vi "Merge Results.vi"(4 "Result 2":T1={"Id"="", "Score"={"Status"=enum."Passed", "cpu_time"=-1, "max_memory"=-1, "style_score"=-1, "score0"="", "score1"="", "score2"="", "score3"="", "score4"="", "score5"=""}}, 5 "Results 1":T1={"Id"="", "Score"={"Status"=enum."Passed", "cpu_time"=-1, "max_memory"=-1, "style_score"=-1, "score0"="", "score1"="", "score2"="", "score3"="", "score4"="", "score5"=""}}) -> (1 "Results":T1={"Id"="", "Score"={"Status"=enum."Passed", "cpu_time"=-1, "max_memory"=-1, "style_score"=-1, "score0"="", "score1"="", "score2"="", "score3"="", "score4"="", "score5"=""}})   [LabVIEW 2013, in "VIChallenge.lvlib"]
doc: "This VI merges two results by selecting the worst case status, adding CPU times, selecting worst case memory usage, worst style score and concatenating custom score fields."
uses:
  <vilib>/LabVIEW Hacker/VIChallenge/VIChallenge.lvlib
  <vilib>/LabVIEW Hacker/VIChallenge/Private/Grader/Type Defs/Grader Result.ctl
  <vilib>/LabVIEW Hacker/VIChallenge/Private/Type Defs/Database/Score.ctl
  <vilib>/LabVIEW Hacker/VIChallenge/Private/Grader/Type Defs/UTF Status.ctl
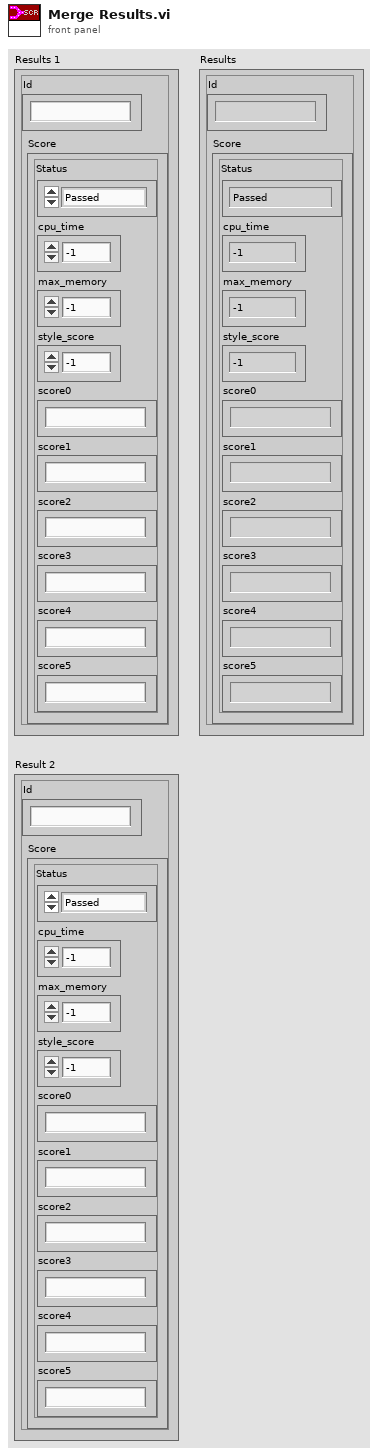
[diagram p1: front panel]
types:
  T1 = typedef "VIChallenge.lvlib/Grader Result.ctl" = cluster{"Id":string, "Score":T2}
  T2 = typedef "VIChallenge.lvlib/Score.ctl" = cluster{"Status":T3, "cpu_time":i32, "max_memory":i32, "style_score":i32, "score0":string, "score1":string, "score2":string, "score3":string, "score4":string, "score5":string}
  T3 = typedef "VIChallenge.lvlib/UTF Status.ctl" = enum16{"Null", "Passed", "Failed", "Error", "Skipped", "Not Processed"}
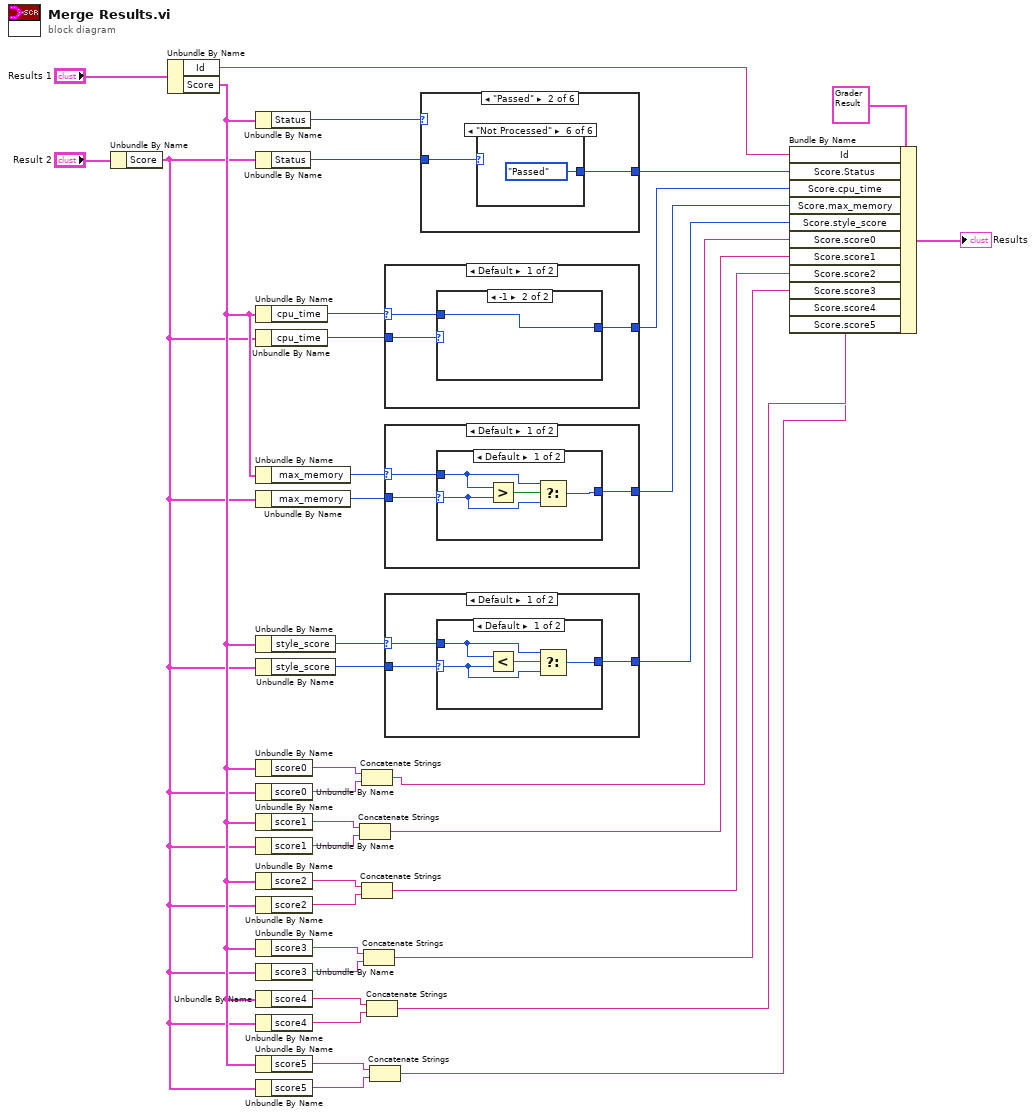
[diagram p0: block diagram]
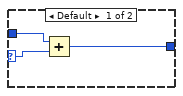
[diagram p6: hidden frame]
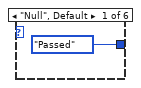
[diagram p9: hidden frame]
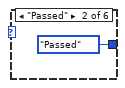
[diagram p10: hidden frame]
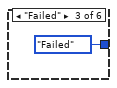
[diagram p11: hidden frame]
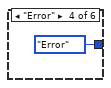
[diagram p12: hidden frame]
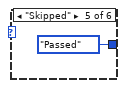
[diagram p13: hidden frame]
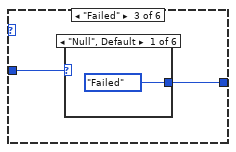
[diagram p14: hidden frame]
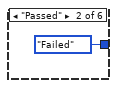
[diagram p15: hidden frame]
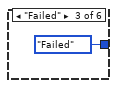
[diagram p16: hidden frame]
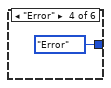
[diagram p17: hidden frame]
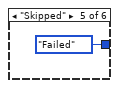
[diagram p18: hidden frame]
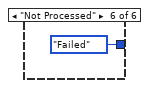
[diagram p19: hidden frame]
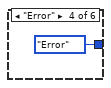
[diagram p20: hidden frame]
diagram:
  n1 = Unbundle By Name("Result 2") -> ("Score"=w14:T2)
  n2 = Unbundle By Name("Results 1") -> ("Id"=w35:string, "Score"=w15:T2)
  n3 = Unbundle By Name(w15) -> ("Status"=w34:T3)
  n4 = Unbundle By Name(w14) -> ("Status"=w32:T3)
  n5 = Unbundle By Name(w15) -> ("cpu_time"=w7:i32)
  n6 = Unbundle By Name(w14) -> ("cpu_time"=w29:i32)
  n7 = Unbundle By Name(w15) -> ("max_memory"=w5:i32)
  n8 = Unbundle By Name(w14) -> ("max_memory"=w4:i32)
  n9 = Unbundle By Name(w15) -> ("style_score"=w3:i32)
  n10 = Unbundle By Name(w14) -> ("style_score"=w2:i32)
  n11 = Unbundle By Name(w15) -> ("score0"=w28:string)
  n12 = Unbundle By Name(w14) -> ("score0"=w27:string)
  n13 = Unbundle By Name(w15) -> ("score1"=w24:string)
  n14 = Unbundle By Name(w14) -> ("score1"=w25:string)
  n15 = Unbundle By Name(w15) -> ("score2"=w23:string)
  n16 = Unbundle By Name(w14) -> ("score2"=w22:string)
  n17 = Unbundle By Name(w15) -> ("score3"=w20:string)
  n18 = Unbundle By Name(w14) -> ("score3"=w21:string)
  n19 = Unbundle By Name(w15) -> ("score4"=w19:string)
  n20 = Unbundle By Name(w14) -> ("score4"=w18:string)
  n21 = Unbundle By Name(w15) -> ("score5"=w16:string)
  n22 = Unbundle By Name(w14) -> ("score5"=w17:string)
  n23 = Concatenate Strings(w24, w25) -> (w13:string)
  n24 = Concatenate Strings(w28, w27) -> (w26:string)
  n25 = Concatenate Strings(w23, w22) -> (w12:string)
  n26 = Concatenate Strings(w20, w21) -> (w11:string)
  n27 = Concatenate Strings(w19, w18) -> (w10:string)
  n28 = Concatenate Strings(w16, w17) -> (w9:string)
  n29 = case shown="Default" w7 {
    selector: w7 -> [w38 _]
    tunnel: [w39 w45] -> w30
    tunnel: w29 -> [w40 w45]
    frame Default {
      n30 = case shown="-1" w40 {
        selector: w40 -> [w42 _]
        tunnel: [w41 w44] -> w39
        tunnel: w38 -> [w43 w44]
        frame Default {
          n31 = Add(x=w43, y=w42) -> (x+y=w41:i32)
        }
        frame -1 {
        }
      }
    }
    frame -1 {
    }
  }
  n32 = case shown="Default" w5 {
    selector: w5 -> [w46 _]
    tunnel: [w47 w54] -> w6
    tunnel: w4 -> [w48 w54]
    frame Default {
      n33 = case shown="Default" w48 {
        selector: w48 -> [w51 _]
        tunnel: [w50 w53] -> w47
        tunnel: w46 -> [w49 w53]
        frame Default {
          n34 = Greater?(x=w49, y=w51) -> (0:w52:bool)
          n35 = Select(t=w49, s=w52, f=w51) -> (s? t:f=w50:i32)
        }
        frame -1 {
        }
      }
    }
    frame -1 {
    }
  }
  n36 = case shown="Default" w3 {
    selector: w3 -> [w55 _]
    tunnel: [w56 w63] -> w1
    tunnel: w2 -> [w57 w63]
    frame Default {
      n37 = case shown="Default" w57 {
        selector: w57 -> [w60 _]
        tunnel: [w59 w62] -> w56
        tunnel: w55 -> [w58 w62]
        frame Default {
          n38 = Less?(x=w58, y=w60) -> (x < y?=w61:bool)
          n39 = Select(t=w58, s=w61, f=w60) -> (s? t:f=w59:i32)
        }
        frame -1 {
        }
      }
    }
    frame -1 {
    }
  }
  n40 = case shown="\"Passed\"" w34 {
    tunnel: w32 -> [w64 w66 w74 _ w82 w83]
    tunnel: [w64 w65 w73 UTF_Status."Error" ("Status") w82 w83] -> w31
    frame "Null", Default {
    }
    frame "Passed" {
      n41 = case shown="\"Not Processed\"" w66 {
        tunnel: [UTF_Status."Passed" ("Status") UTF_Status."Passed" ("Status") UTF_Status."Failed" ("Status") UTF_Status."Error" ("Status") UTF_Status."Passed" ("Status") UTF_Status."Passed" ("Status")] -> w65
        frame "Null", Default {
        }
        frame "Passed" {
        }
        frame "Failed" {
        }
        frame "Error" {
        }
        frame "Skipped" {
        }
        frame "Not Processed" {
        }
      }
    }
    frame "Failed" {
      n42 = case shown="\"Null\", Default" w74 {
        tunnel: [UTF_Status."Failed" ("Status") UTF_Status."Failed" ("Status") UTF_Status."Failed" ("Status") UTF_Status."Error" ("Status") UTF_Status."Failed" ("Status") UTF_Status."Failed" ("Status")] -> w73
        frame "Null", Default {
        }
        frame "Passed" {
        }
        frame "Failed" {
        }
        frame "Error" {
        }
        frame "Skipped" {
        }
        frame "Not Processed" {
        }
      }
    }
    frame "Error" {
    }
    frame "Skipped" {
    }
    frame "Not Processed" {
    }
  }
  n43 = Bundle By Name(cluster=T1 {"Id"="", "Score"={"Status"=enum."Passed", "cpu_time"=-1, "max_memory"=-1, "style_score"=-1, "score0"="", "score1"="", "score2"="", "score3"="", "score4"="", "score5"=""}} ("Results 1"), "Id"=w35, "Score.Status"=w31, "Score.cpu_time"=w30, "Score.max_memory"=w6, "Score.style_score"=w1, "Score.score0"=w26, "Score.score1"=w13, "Score.score2"=w12, "Score.score3"=w11, "Score.score4"=w10, "Score.score5"=w9) -> (→"Results":T1)
